vi "CallOutputList.vi"(5 "list":string, 9 "Function in":refnum<class "Function.lvclass">) -> (3 "Function out":refnum<class "Function.lvclass">, 4 "call outputs":string)   [LabVIEW 2014, in "Raspberry Pi Compatible Compiler for LabVIEW.lvlib" / "Function.lvclass"]
uses:
  Function.lvclass
  Python/Parsing/ListTypesTD.ctl
  Terminal/Terminal.lvclass
  Python/Parsing/Python Functions.lvlib
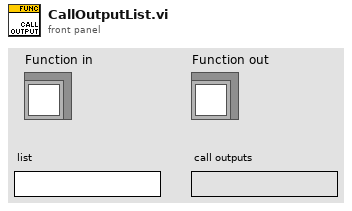
[diagram p1: front panel]
types:
  T1 = typedef "Raspberry Pi Compatible Compiler for LabVIEW.lvlib/Python Functions.lvlib/ListTypesTD.ctl" = enum16{"list", "tuple", "parameter list", "output list", "return values"}
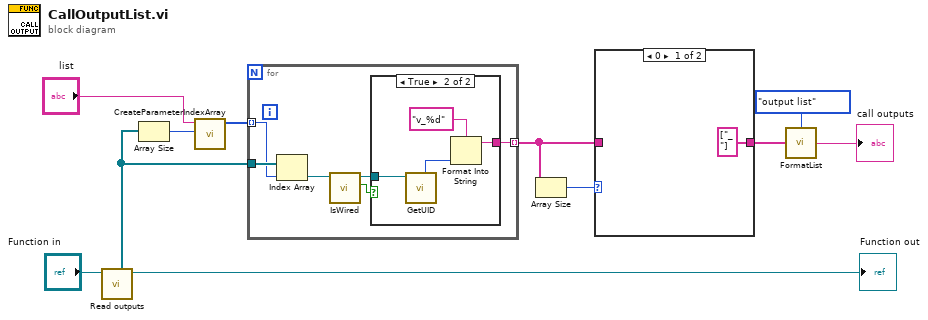
[diagram p0: block diagram]
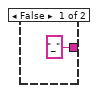
[diagram p3: hidden frame]
diagram:
  n1 = call-dynamic "Read outputs.vi"("Node in"="Function in") -> ("Node out"=→"Function out":refnum<class "Function.lvclass">, "outputs"=w3:refnum<class "Terminal.lvclass">[])  [unwired: 7 in]
  n2 = Array Size(array=w3) -> (size(s)=w11:i32)
  n3 = call "CreateParameterIndexArray.vi"("length"=w11, "list"="list") -> ("Array"=w10:i32[])  [unwired: 9 in]
  n4 = for {
    tunnel: w10 -> [w16] mode=indexing
    tunnel: w3 -> [w17]
    tunnel: [w15] -> w7 mode=indexing
    n5 = Index Array(array=w17, index=w16) -> (element=w14:refnum<class "Terminal.lvclass">)
    n6 = call "IsWired.vi"("Terminal in"=w14) -> ("wired"=w12:bool, "Terminal out"=w13:refnum<class "Terminal.lvclass">)  [unwired: 6 in, 1 out]
    n7 = case shown="True" w12 {
      tunnel: ["_" w22] -> w15
      tunnel: w13 -> [_ w20]
      frame False {
      }
      frame True {
        n8 = call-dynamic "GetUID.vi"("GObject in"=w20) -> ("UID"=w19:i32)  [unwired: 6 in, 2 out]
        n9 = Format Into String(format string="v_%d", w19) -> (resulting string=w22:string)  [unwired: 2 in, 1 out]
      }
    }
  }
  n10 = Array Size(array=w7) -> (size(s)=w8:i32)
  n11 = case shown="0" w8 {
    tunnel: w7 -> [_ w24]
    tunnel: [string[] ["_"] w24] -> w6
    frame 0 {
    }
    frame Default {
    }
  }
  n12 = call "FormatList.vi"("values"=w6, "type"=ListTypesTD."output list") -> ("python object"=→"call outputs":string)
